vi "Control & Mapping.vi"() -> ()   [LabVIEW 2015]
uses:
  <vilib>/Instr/_visa.llb/VISA Configure Serial Port (Instr).vi
  <vilib>/Utility/inputDevices.llb/keyboardAcquire.vi
  <vilib>/Utility/inputDevices.llb/closeKeyboard.vi
panel:
  in  "path to PNG file":path
  out "Metres Travelled":dbl
  out "From Xbee":string
  out "Metal Sensors":string
  out "yplot2":dbl
  out "xplot2":dbl
  out "yplot1":dbl
  out "xplot1":dbl
  out "Right MS":bool
  out "Left MS":bool
  out "hi":dbl
  out "Y":dbl
  out "X":dbl
  in  "Direction in the Field":dbl
  out "TR":bool
  out "TL":bool
  out "MAP (19x19)":picture
  out "R":bool
  out "B":bool
  out "L":bool
  out "F":bool
  out "To Xbee":string
  in  "Required Speed":dbl=1.0 min=1.0 max=3.0 step=1.0
  # "Note:\n1 --> Low Speed\n2 --> Medium Speed\n3 --> High Speed"
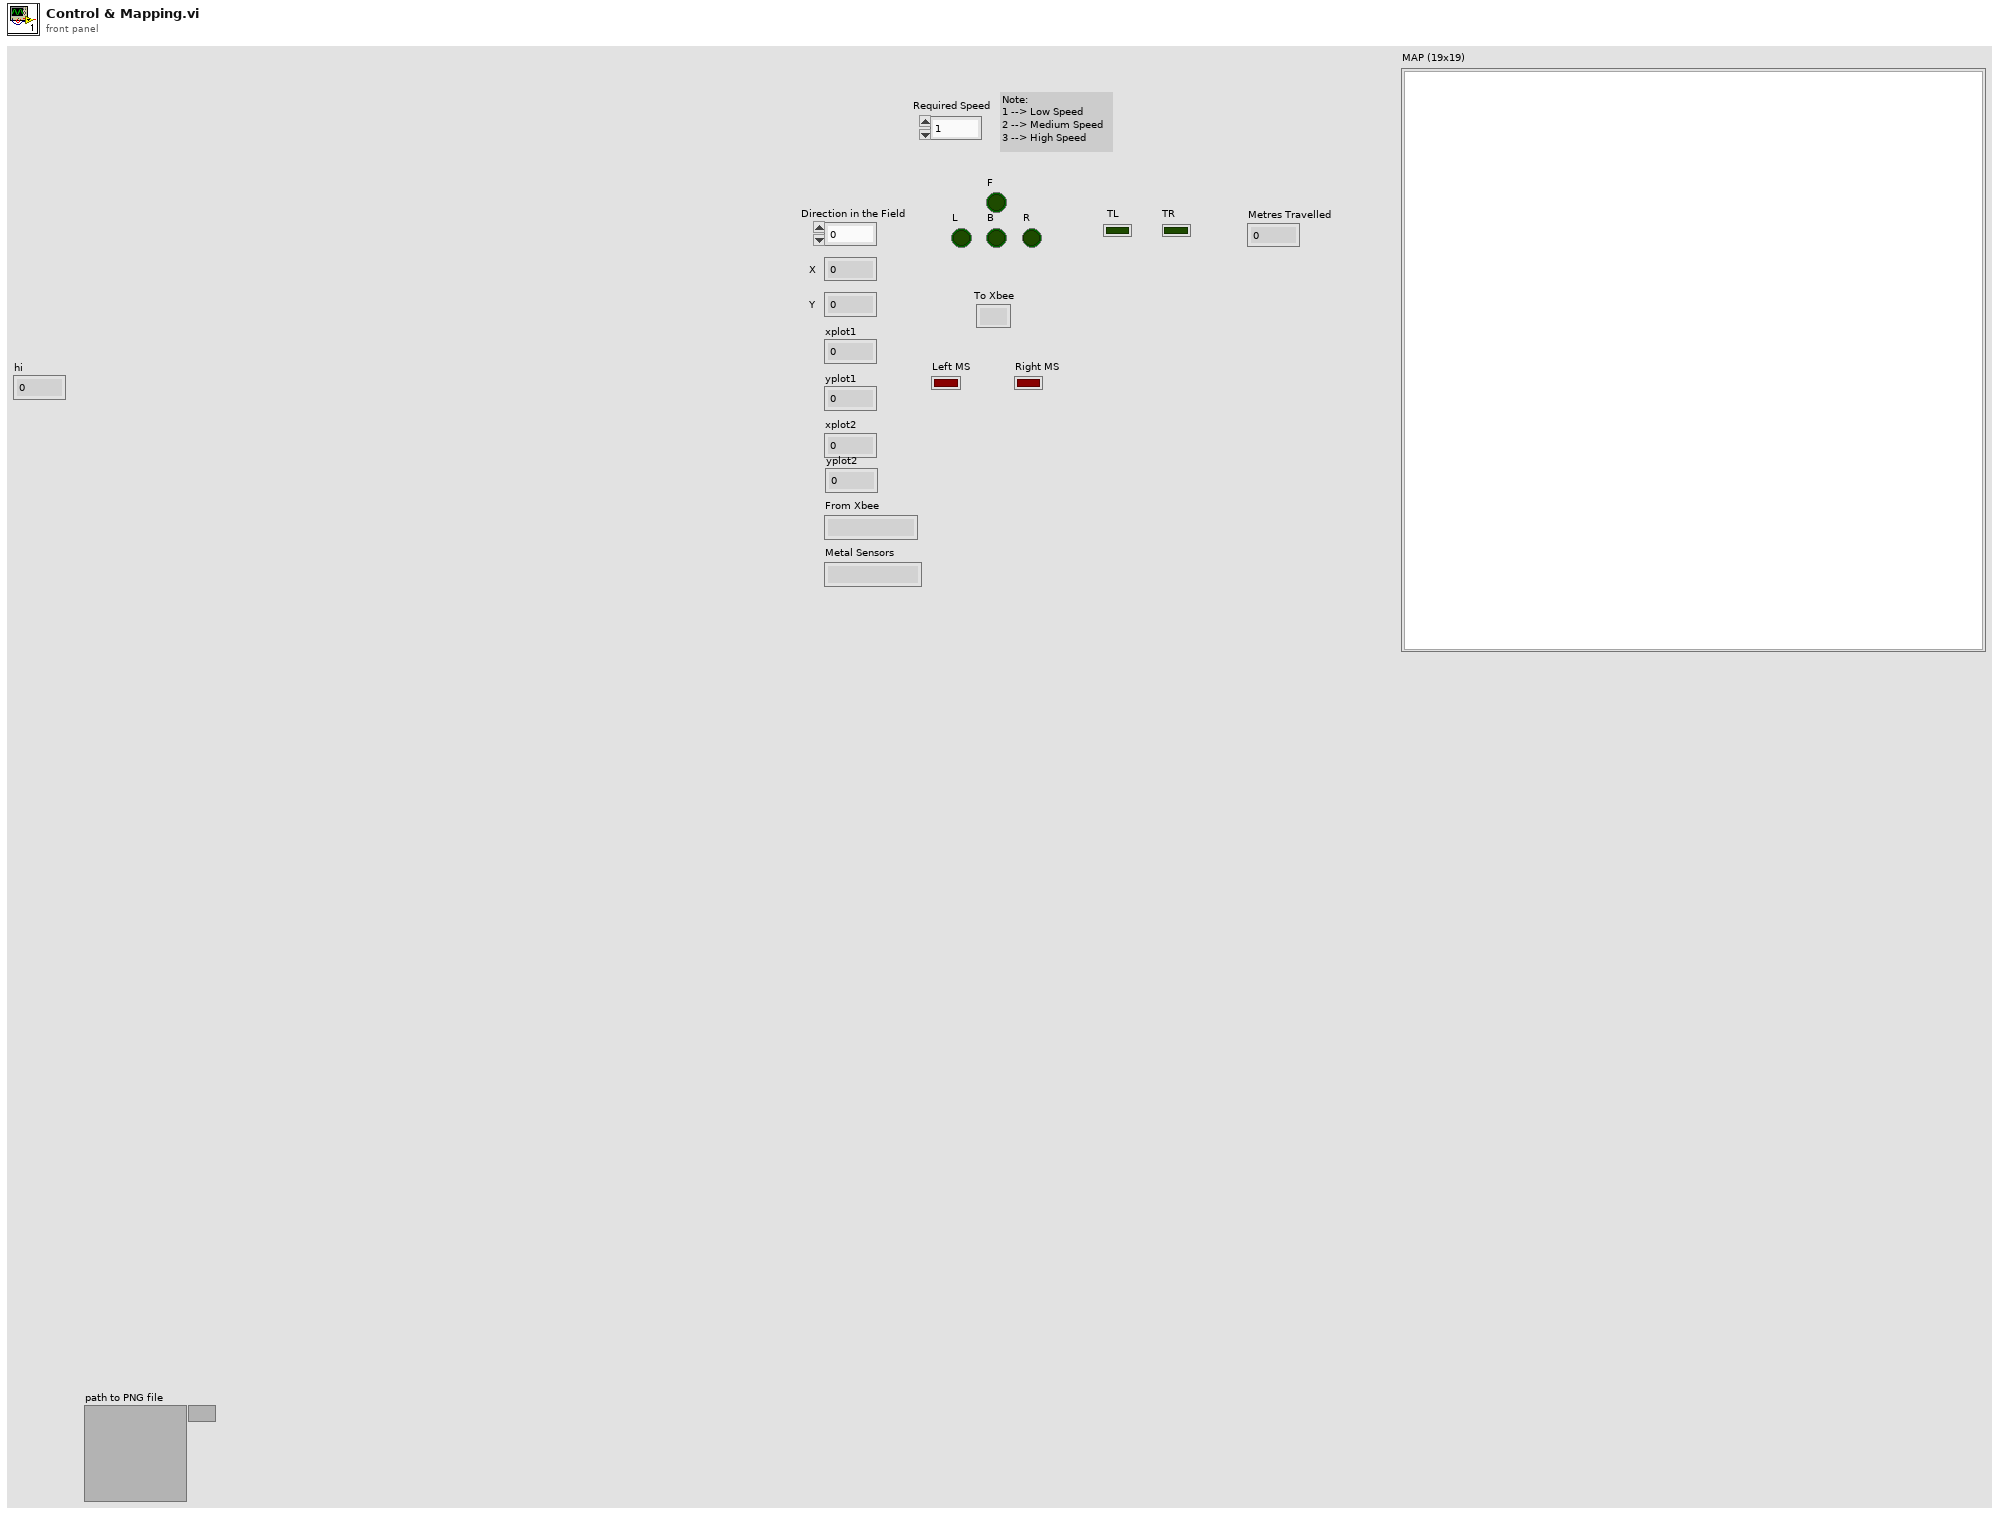
[diagram p1: front panel]
types:
  T1 = typedef "imagedata.ctl" = cluster{"image type":i32, "image depth":i32, "image":u8[], "mask":u8[], "colors":u32[], "Rectangle":cluster{"left":i16, "top":i16, "right":i16, "bottom":i16}}
  T2 = cluster{"Width":u16, "Style":enum32{"Solid", "Dash", "Dot", "DashDot", "DashDotDot"}}
  T3 = enum16{"0", "1", "2", "3", "4", "5", "6", "7", "8", "9", "A", "B", "C", "D", "E", "F", "G", "H", "I", "J", "K", "L", "M", "N", "O", "P", "Q", "R", "S", "T", "U", "V", "W", "X", "Y", "Z", "F1", "F2", "F3", "F4", "F5", "F6", "F7", "F8", "F9", "F10", "F11", "F12", "F13", "F14", "F15", "ADD", "BACK", "BACKSLASH", "CAPITAL", "COMMA", "DECIMAL", "DELETE", "DIVIDE", "DOWN", "END", "EQUALS", "ESCAPE", "GRAVE (`)", "HOME", "INSERT", "LBRACKET", "LCONTROL", "LEFT", "L ALT", "LSHIFT", "LWIN", "MINUS", "MULTIPLY", "NEXT", "NUMLOCK", "NUMPAD_0", "NUMPAD_1", "NUMPAD_2", "NUMPAD_3", "NUMPAD_4", "NUMPAD_5", "NUMPAD_6", "NUMPAD_7", "NUMPAD_8", "NUMPAD_9", "PAUSE", "PERIOD", "PRIOR (PG UP)", "RBRACKET", "RCONTROL", "RETURN", "RIGHT", "R ALT", "RSHIFT", "RWIN", "SCROLL", "SEMICOLON", "SLASH", "SPACE", "SUBTRACT", "TAB", "UP", "ENTER (num pad)", "' (quote)"}[]
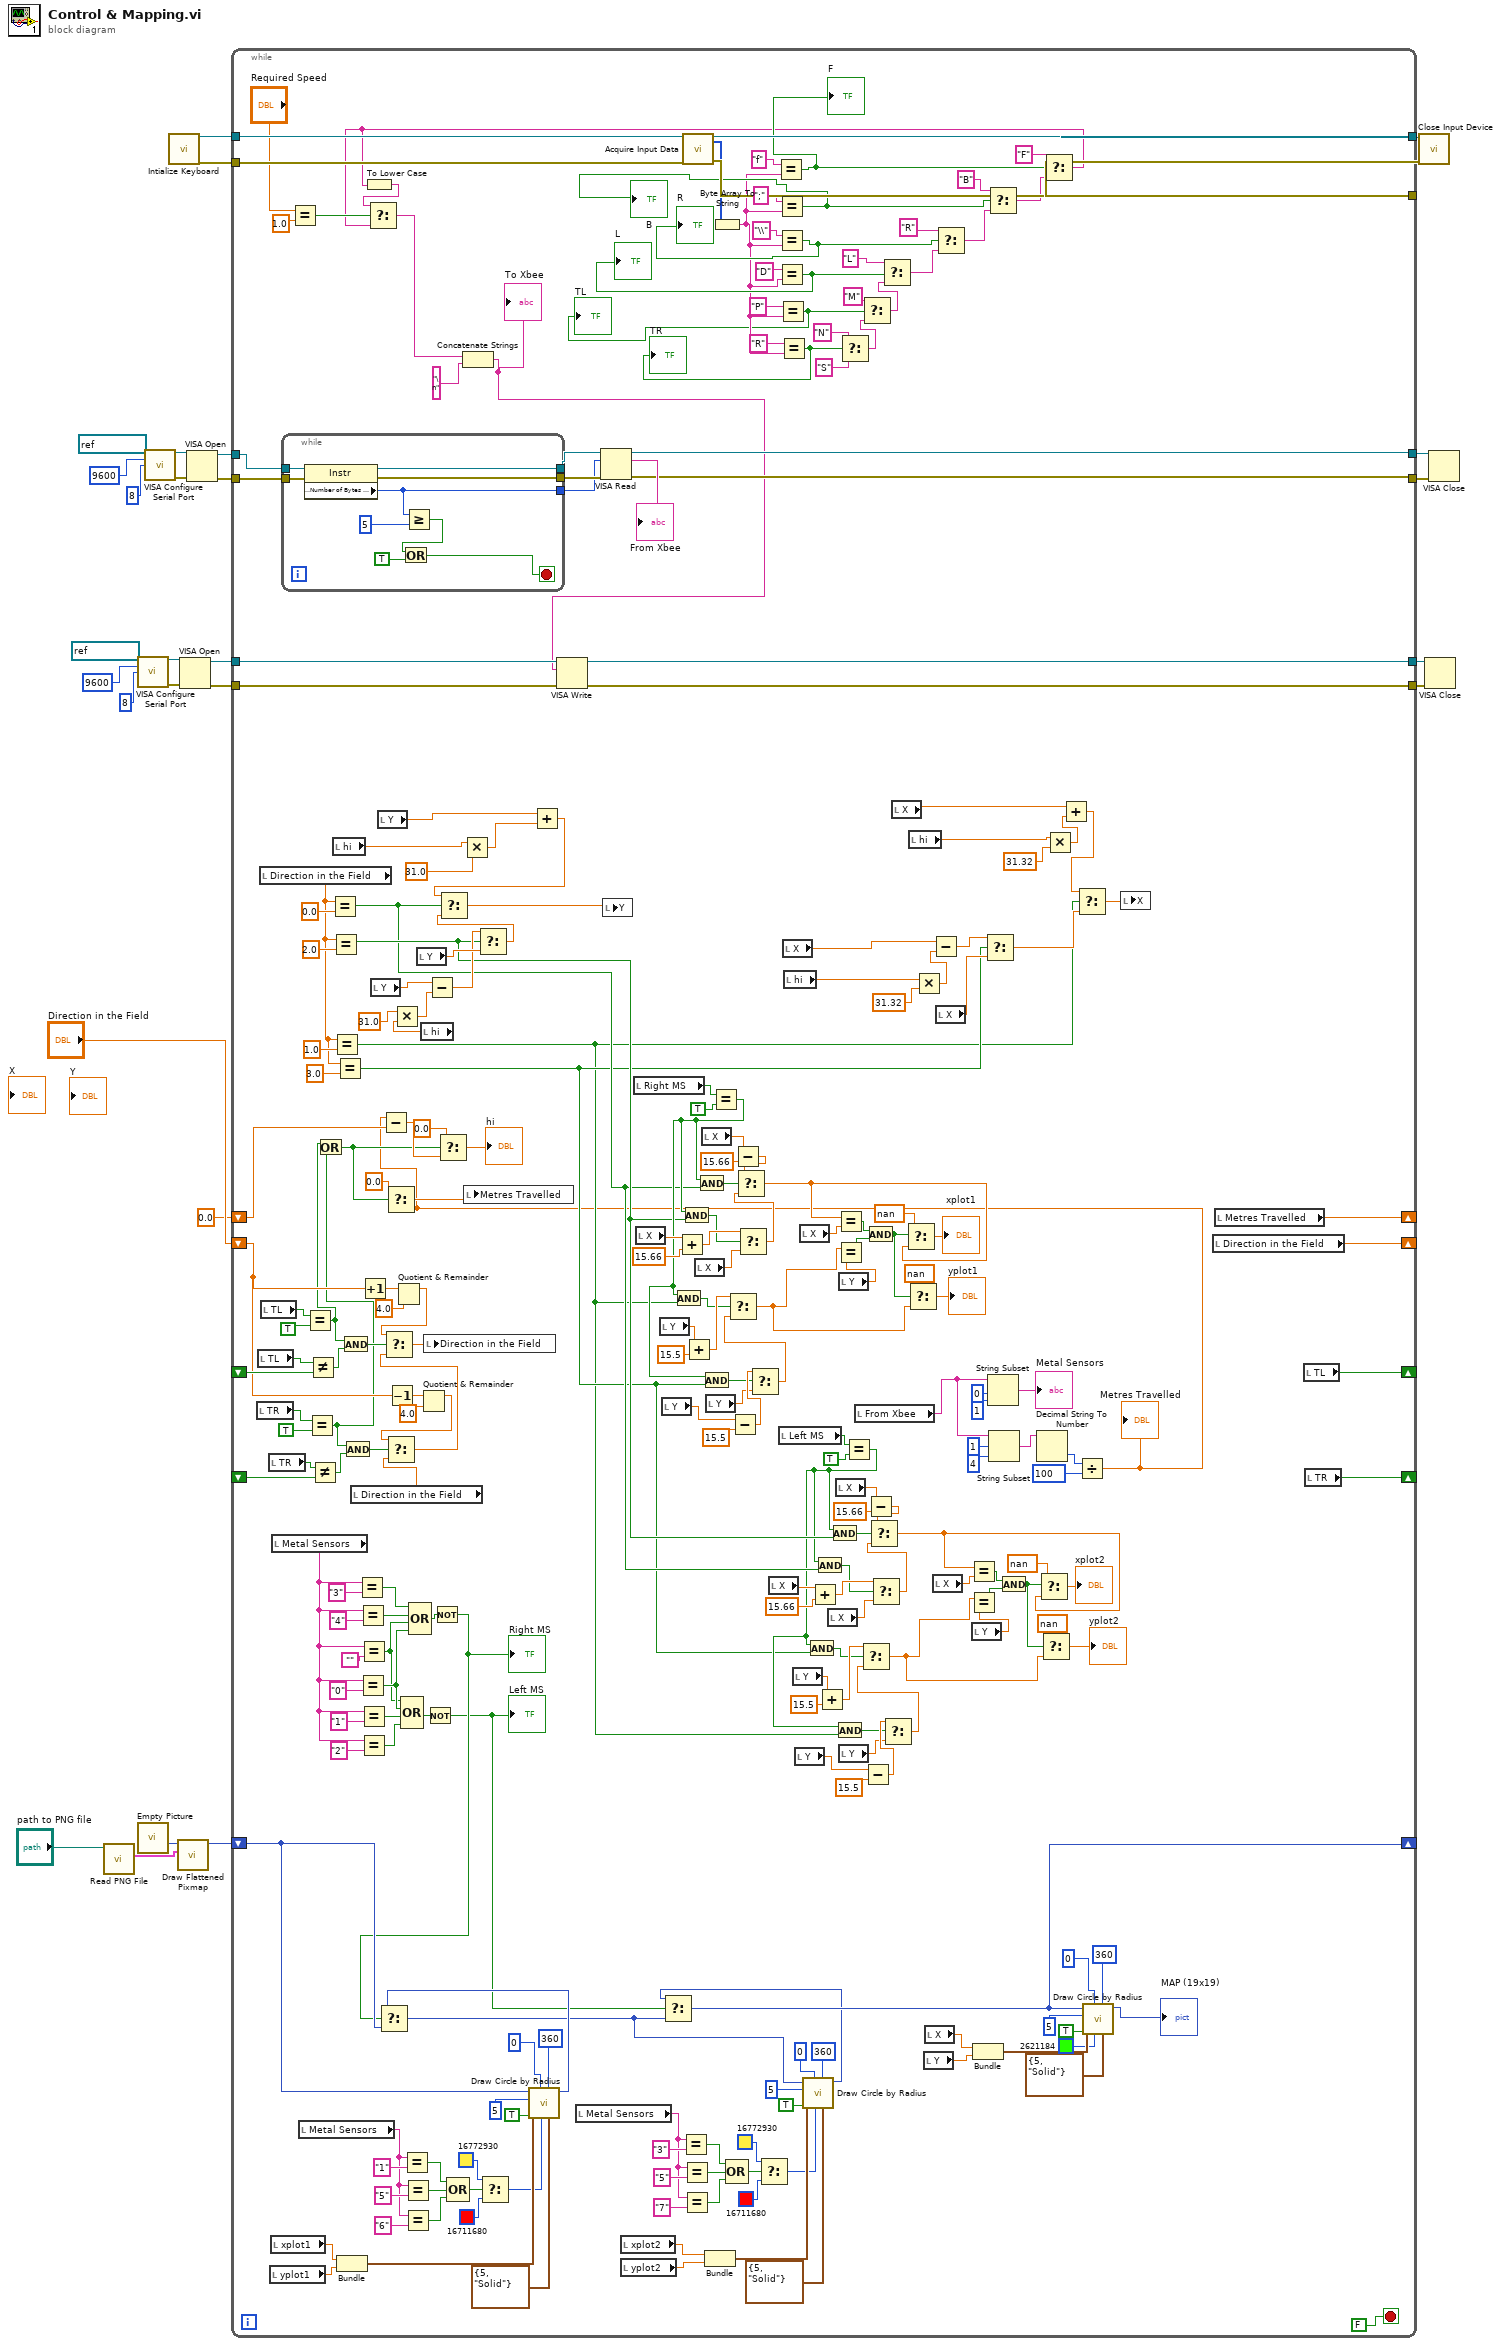
[diagram p0: block diagram]
diagram:
  n1 = call <vilib>:"Read PNG File.vi"("path to PNG file"="path to PNG file") -> ("image data"=w12:T1)  [unwired: 8 in, 2 out]
  n2 = call-poly "VISA Configure Serial Port"("VISA resource name"=refnum<visa-resource-name> "COM10", "baud rate (9600)"=u32 9600, "data bits (8)"=u16 8) -> ("VISA resource name out"=w9:refnum<visa-resource-name>, "error out"=w8:errorcluster)  [unwired: 11 in]
  n3 = call "Empty Picture"() -> ("empty picture"=w13:picture)
  n4 = call-poly "VISA Configure Serial Port"("VISA resource name"=refnum<visa-resource-name> "COM12", "baud rate (9600)"=u32 9600, "data bits (8)"=u16 8) -> ("VISA resource name out"=w20:refnum<visa-resource-name>, "error out"=w19:errorcluster)  [unwired: 11 in]
  n5 = call <vilib>:"Intialize Keyboard.vi"() -> ("error out"=w27:errorcluster, "device ID"=w28:refnum<k1>)  [unwired: 10 in]
  n6 = call <vilib>:"Draw Flattened Pixmap.vi"("image data"=w12, "picture"=w13) -> ("new picture"=w10:picture)  [unwired: 7 in]
  n7 = VISA Open(error in (no error)=w8, VISA resource name=w9) -> (VISA resource name=w4:refnum<visa-resource-name>, error out=w3:errorcluster)  [unwired: 3 in]
  n8 = VISA Open(error in (no error)=w19, VISA resource name=w20) -> (VISA resource name=w24:refnum<visa-resource-name>, error out=w21:errorcluster)  [unwired: 3 in]
  n9 = while {
    tunnel: w28 -> [w297]
    tunnel: w27 -> [w296]
    tunnel: [w295] -> w26
    tunnel: [w294] -> w25
    tunnel: w24 -> [w46]
    tunnel: [w35] -> w23
    tunnel: [w34] -> w22
    tunnel: w21 -> [w44]
    shift-right: [w226] -> _
    shift-left: 0.0 ("Metres Travelled (From Encoder)") -> [w197]
    shift-right: [w225] -> _
    shift-left: "Direction in the Field" -> [w202]
    shift-right: [w224] -> _
    shift-left: _ -> [w219]
    shift-right: [w223] -> _
    shift-left: _ -> [w211]
    shift-right: [w109] -> _
    shift-left: w10 -> [w165]
    tunnel: w4 -> [w33]
    tunnel: w3 -> [w32]
    tunnel: [w31] -> w2
    tunnel: [w30] -> w1
    stop <- FALSE stop-if-true
    n10 = local read "TR"() -> (w210:bool)
    n11 = local read "TL"() -> (w220:bool)
    n12 = local read "Direction in the Field"() -> (w231:dbl)
    n13 = local read "TL"() -> (w222:bool)
    n14 = local read "TR"() -> (w208:bool)
    n15 = local read "yplot1"() -> (w163:dbl)
    n16 = local read "xplot1"() -> (w162:dbl)
    n17 = local read "Metal Sensors"() -> (w40:string)
    n18 = while {
      tunnel: [w306] -> w43
      tunnel: w46 -> [w304]
      tunnel: [w303] -> w45
      tunnel: w44 -> [w302]
      tunnel: [w301] -> w42
      stop <- w298 stop-if-true
      n19 = property class="Instr"(reference=w304, error in=w302) -> (reference out=w303:refnum<visa-resource-name>, error out=w306:errorcluster, "Serial Settings:Number of Bytes at Serial Port"=w301:u32)
      n20 = Greater Or Equal?(x=w301, y=u32 5) -> (x >= y?=w300:bool)
      n21 = Or(x=w300, y=TRUE) -> (x .or. y?=w298:bool)
    }
    n22 = Equal?(x="Required Speed", y=1.0) -> (x = y?=w50:bool)
    n23 = local read "Metal Sensors"() -> (w81:string)
    n24 = Equal?(x=w222, y=TRUE) -> (x = y?=w36:bool)
    n25 = Equal?(x=w210, y=TRUE) -> (x = y?=w200:bool)
    n26 = Not Equal?(x=w220, y=w219) -> (x != y?=w218:bool)
    n27 = Not Equal?(x=w208, y=w211) -> (x != y?=w212:bool)
    n28 = Or(x=w36, y=w200) -> (x .or. y?=w195:bool)
    n29 = Equal?(x=w231, y=0.0) -> (x = y?=w113:bool)
    n30 = Equal?(x=w231, y=2.0) -> (x = y?=w114:bool)
    n31 = Equal?(x=w231, y=1.0) -> (x = y?=w110:bool)
    n32 = local read "hi"() -> (w253:dbl)
    n33 = Equal?(x=w231, y=3.0) -> (x = y?=w111:bool)
    n34 = Bundle("xplot1"=w162, "yplot1"=w163) -> (w171:cluster{"xplot1":dbl, "yplot1":dbl})  [unwired: 1 in]
    n35 = And(x=w36, y=w218) -> (x .and. y?=w217:bool)
    n36 = And(x=w200, y=w212) -> (x .and. y?=w207:bool)
    n37 = local read "Direction in the Field"() -> (w203:dbl)
    n38 = Equal?(x=w40, y="3") -> (x = y?=w95:bool)
    n39 = Equal?(x=w40, y="4") -> (x = y?=w94:bool)
    n40 = Equal?(x=w40, y="0") -> (x = y?=w41:bool)
    n41 = Equal?(x=w40, y="") -> (x = y?=w38:bool)
    n42 = Equal?(x=w40, y="1") -> (x = y?=w90:bool)
    n43 = Equal?(x=w40, y="2") -> (x = y?=w89:bool)
    n44 = Increment(x=w202) -> (x+1=w216:dbl)
    n45 = local read "Y"() -> (w236:dbl)
    n46 = local read "Y"() -> (w254:dbl)
    n47 = Decrement(x=w202) -> (x-1=w206:dbl)
    n48 = Quotient & Remainder(x=w216, y=4.0) -> (x-y*floor(x/y)=w214:dbl)  [unwired: 1 out]
    n49 = Compound Arithmetic op=OR(w38, w41, w90, w89) -> (w88:bool)
    n50 = Equal?(x=w81, y="1") -> (x = y?=w84:bool)
    n51 = Equal?(x=w81, y="5") -> (x = y?=w83:bool)
    n52 = Equal?(x=w81, y="6") -> (x = y?=w82:bool)
    n53 = Compound Arithmetic op=OR(w95, w94, w38, w41) -> (w93:bool)
    n54 = local read "Y"() -> (w235:dbl)
    n55 = Quotient & Remainder(x=w206, y=4.0) -> (x-y*floor(x/y)=w204:dbl)  [unwired: 1 out]
    n56 = Select(t=w204, s=w207, f=w203) -> (s? t:f=w201:dbl)
    n57 = Select(t=w214, s=w217, f=w201) -> (s? t:f=w213:dbl)
    n58 = local read "hi"() -> (w251:dbl)
    n59 = Multiply(x=31.0 ("y"), y=w251) -> (x*y=w249:dbl)
    n60 = local write "Direction in the Field"(w213) -> ()
    n61 = Not(x=w88) -> (.not. x?=w64:bool)
    "Left MS" <- w64
    n62 = Subtract(x=w236, y=w249) -> (x-y=w234:dbl)
    n63 = Not(x=w93) -> (.not. x?=w65:bool)
    "Right MS" <- w65
    n64 = Compound Arithmetic op=OR(w84, w83, w82) -> (w80:bool)
    n65 = Multiply(x=w253, y=31.0) -> (x*y=w252:dbl)
    n66 = Select(t=w234, s=w114, f=w235) -> (s? t:f=w233:dbl)
    n67 = Select(t=u32 16772930 ("color(black)"), s=w80, f=u32 16711680 ("color(black)")) -> (s? t:f=w77:u32)
    n68 = call <vilib>:"Draw Circle by Radius.vi"("pen"=T2 {"Width"=5, "Style"=enum."Solid"}, "arc size(360)"=360, "color(black)"=w77, "start angle(0)"=0, "fill?(F)"=TRUE, "pixel center"=w171, "radius"=i16 5, "picture"=w165) -> ("new picture"=w164:picture)  [unwired: 3 in]
    n69 = Select(t=w164, s=w65, f=w165) -> (s? t:f=w100:picture)
    n70 = Add(x=w254, y=w252) -> (x+y=w255:dbl)
    n71 = Select(t=w255, s=w113, f=w233) -> (s? t:f=w248:dbl)
    n72 = local read "Metal Sensors"() -> (w67:string)
    n73 = VISA Read(VISA resource name=w45, byte count=w42, error in (no error)=w43) -> (VISA resource name out=w35:refnum<visa-resource-name>, read buffer=→"From Xbee":string, error out=w34:errorcluster)  [unwired: 1 out]
    n74 = local write "Y"(w248) -> ()
    n75 = local read "xplot2"() -> (w103:dbl)
    n76 = local read "yplot2"() -> (w102:dbl)
    n77 = local read "Right MS"() -> (w191:bool)
    n78 = local read "X"() -> (w187:dbl)
    n79 = local read "Y"() -> (w181:dbl)
    n80 = local read "Y"() -> (w176:dbl)
    n81 = Add(x=w187, y=15.66) -> (x+y=w185:dbl)
    n82 = Equal?(x=w67, y="3") -> (x = y?=w73:bool)
    n83 = Equal?(x=w67, y="5") -> (x = y?=w72:bool)
    n84 = Equal?(x=w67, y="7") -> (x = y?=w71:bool)
    n85 = call-poly <vilib>:"Acquire Input Data.vi"("device ID"=w297, "error in (no error)"=w296) -> ("device ID"=w295:refnum<k1>, "keys pressed"=w292:T3, "error out"=w294:errorcluster)  [unwired: 15 in]
    n86 = Add(x=w181, y=15.5) -> (x+y=w179:dbl)
    n87 = local read "X"() -> (w161:dbl)
    n88 = local read "X"() -> (w189:dbl)
    n89 = Bundle("xplot2"=w103, "yplot2"=w102) -> (w108:cluster{"xplot2":dbl, "yplot2":dbl})  [unwired: 1 in]
    n90 = local read "Y"() -> (w159:dbl)
    n91 = Equal?(x=w191, y=TRUE) -> (x = y?=w178:bool)
    n92 = And(x=w178, y=w110) -> (x .and. y?=w174:bool)
    n93 = And(x=w178, y=w114) -> (x .and. y?=w182:bool)
    n94 = And(x=w178, y=w113) -> (x .and. y?=w183:bool)
    n95 = And(x=w178, y=w111) -> (x .and. y?=w173:bool)
    n96 = Byte Array To String(unsigned byte array=w292) -> (string=w275:string)
    n97 = Compound Arithmetic op=OR(w73, w72, w71) -> (w70:bool)
    n98 = Subtract(x=w176, y=15.5) -> (x-y=w175:dbl)
    n99 = Subtract(x=w189, y=15.66) -> (x-y=w188:dbl)
    n100 = Select(t=w185, s=w182, f=w161) -> (s? t:f=w184:dbl)
    n101 = Select(t=w188, s=w183, f=w184) -> (s? t:f=w152:dbl)
    n102 = Select(t=w175, s=w173, f=w159) -> (s? t:f=w177:dbl)
    n103 = Select(t=w179, s=w174, f=w177) -> (s? t:f=w149:dbl)
    n104 = Select(t=u32 16772930 ("color(black)"), s=w70, f=u32 16711680 ("color(black)")) -> (s? t:f=w66:u32)
    n105 = local read "X"() -> (w145:dbl)
    n106 = Equal?(x="f", y=w275) -> (x = y?=w279:bool)
    "F" <- w279
    n107 = Equal?(x=";", y=w275) -> (x = y?=w278:bool)
    "B" <- w278
    n108 = Equal?(x="\\", y=w275) -> (x = y?=w277:bool)
    "R" <- w277
    n109 = Equal?(x="D", y=w275) -> (x = y?=w276:bool)
    "L" <- w276
    n110 = Equal?(x="P", y=w275) -> (x = y?=w267:bool)
    "TL" <- w267
    n111 = Equal?(x="R", y=w275) -> (x = y?=w266:bool)
    "TR" <- w266
    n112 = local read "Left MS"() -> (w118:bool)
    n113 = local read "X"() -> (w240:dbl)
    n114 = local read "hi"() -> (w241:dbl)
    n115 = local read "Y"() -> (w139:dbl)
    n116 = local read "Y"() -> (w135:dbl)
    n117 = local read "X"() -> (w156:dbl)
    n118 = call <vilib>:"Draw Circle by Radius.vi"("pen"=T2 {"Width"=5, "Style"=enum."Solid"}, "arc size(360)"=360, "color(black)"=w66, "start angle(0)"=0, "fill?(F)"=TRUE, "pixel center"=w108, "radius"=i16 5, "picture"=w100) -> ("new picture"=w99:picture)  [unwired: 3 in]
    n119 = Select(t=w99, s=w64, f=w100) -> (s? t:f=w109:picture)
    n120 = Add(x=w145, y=15.66) -> (x+y=w143:dbl)
    n121 = Add(x=w139, y=15.5) -> (x+y=w137:dbl)
    n122 = local read "X"() -> (w131:dbl)
    n123 = Equal?(x=w152, y=w156) -> (x = y?=w158:bool)
    n124 = local read "X"() -> (w117:dbl)
    n125 = local read "Y"() -> (w155:dbl)
    n126 = Equal?(x=w149, y=w155) -> (x = y?=w157:bool)
    n127 = local read "Y"() -> (w129:dbl)
    n128 = Select(t="N", s=w266, f="S") -> (s? t:f=w269:string)
    n129 = Equal?(x=w118, y=TRUE) -> (x = y?=w112:bool)
    n130 = And(x=w112, y=w111) -> (x .and. y?=w133:bool)
    n131 = And(x=w112, y=w113) -> (x .and. y?=w140:bool)
    n132 = And(x=w112, y=w114) -> (x .and. y?=w141:bool)
    n133 = And(x=w112, y=w110) -> (x .and. y?=w132:bool)
    n134 = local read "From Xbee"() -> (w55:string)
    n135 = Select(t="M", s=w267, f=w269) -> (s? t:f=w270:string)
    n136 = Subtract(x=w135, y=15.5) -> (x-y=w134:dbl)
    n137 = And(x=w158, y=w157) -> (x .and. y?=w151:bool)
    n138 = Subtract(x=w117, y=15.66) -> (x-y=w146:dbl)
    n139 = Select(t=w143, s=w140, f=w131) -> (s? t:f=w142:dbl)
    n140 = Select(t=w146, s=w141, f=w142) -> (s? t:f=w123:dbl)
    n141 = Select(t="L", s=w276, f=w270) -> (s? t:f=w285:string)
    n142 = Select(t=w134, s=w132, f=w129) -> (s? t:f=w136:dbl)
    n143 = Select(t=w137, s=w133, f=w136) -> (s? t:f=w120:dbl)
    n144 = local read "X"() -> (w244:dbl)
    n145 = Select(t=nan, s=w151, f=w152) -> (s? t:f=→"xplot1":dbl)
    n146 = Select(t=nan, s=w151, f=w149) -> (s? t:f=→"yplot1":dbl)
    n147 = local read "hi"() -> (w247:dbl)
    n148 = Multiply(x=w241, y=31.32) -> (x*y=w229:dbl)
    n149 = local read "Y"() -> (w237:dbl)
    n150 = local read "X"() -> (w238:dbl)
    n151 = Subtract(x=w240, y=w229) -> (x-y=w230:dbl)
    n152 = local read "X"() -> (w126:dbl)
    n153 = Select(t="R", s=w277, f=w285) -> (s? t:f=w287:string)
    n154 = local read "X"() -> (w228:dbl)
    n155 = Equal?(x=w123, y=w126) -> (x = y?=w128:bool)
    n156 = local read "Y"() -> (w125:dbl)
    n157 = Equal?(x=w120, y=w125) -> (x = y?=w127:bool)
    n158 = Bundle("X"=w238, "Y"=w237) -> (w265:cluster{"X":dbl, "Y":dbl})  [unwired: 1 in]
    n159 = Select(t=w230, s=w111, f=w228) -> (s? t:f=w227:dbl)
    n160 = Select(t="B", s=w278, f=w287) -> (s? t:f=w286:string)
    n161 = String Subset(string=w55, offset (0)=0, length (rest)=1 ("length (rest)")) -> (substring=→"Metal Sensors":string)
    n162 = String Subset(string=w55, offset (0)=1, length (rest)=4 ("length (rest)")) -> (substring=w58:string)
    n163 = And(x=w128, y=w127) -> (x .and. y?=w122:bool)
    n164 = Decimal String To Number(string=w58) -> (number=w57:i32)  [unwired: 2 in, 1 out]
    n165 = Select(t=nan, s=w122, f=w123) -> (s? t:f=→"xplot2":dbl)
    n166 = Select(t=nan, s=w122, f=w120) -> (s? t:f=→"yplot2":dbl)
    n167 = Select(t="F", s=w279, f=w286) -> (s? t:f=w48:string)
    n168 = To Lower Case(string=w48) -> (all lower case string=w49:string)
    n169 = Select(t=w49, s=w50, f=w48) -> (s? t:f=w47:string)
    n170 = Concatenate Strings(w47, "\n" ("string")) -> (w29:string)
    "To Xbee" <- w29
    n171 = VISA Write(VISA resource name=w33, write buffer=w29, error in (no error)=w32) -> (VISA resource name out=w31:refnum<visa-resource-name>, error out=w30:errorcluster)  [unwired: 1 out]
    n172 = Multiply(x=w247, y=31.32) -> (x*y=w245:dbl)
    n173 = Add(x=w244, y=w245) -> (x+y=w243:dbl)
    n174 = Select(t=w243, s=w110, f=w227) -> (s? t:f=w239:dbl)
    n175 = Divide(x=w57, y=100) -> (x/y=w37:dbl)
    "Metres Travelled" <- w37
    n176 = Subtract(x=w37, y=w197) -> (x-y=w196:dbl)
    n177 = Select(t=0.0, s=w195, f=w37) -> (s? t:f=w193:dbl)
    n178 = Select(t=0.0, s=w195, f=w196) -> (s? t:f=→"hi":dbl)
    n179 = local write "Metres Travelled"(w193) -> ()
    n180 = call <vilib>:"Draw Circle by Radius.vi"("pen"=T2 {"Width"=5, "Style"=enum."Solid"}, "arc size(360)"=360, "color(black)"=u32 2621184, "start angle(0)"=0, "fill?(F)"=TRUE, "pixel center"=w265, "radius"=i16 5, "picture"=w109) -> ("new picture"=→"MAP (19x19)":picture)  [unwired: 3 in]
    n181 = local write "X"(w239) -> ()
    n182 = local read "Direction in the Field"() -> (w225:dbl)
    n183 = local read "Metres Travelled"() -> (w226:dbl)
    n184 = local read "TL"() -> (w224:bool)
    n185 = local read "TR"() -> (w223:bool)
  }
  n186 = call-poly <vilib>:"Close Input Device.vi"("error in (no error)"=w25, "device ID"=w26) -> ()  [unwired: 8 in, 1 out]
  n187 = VISA Close(VISA resource name=w2, error in (no error)=w1) -> ()  [unwired: 1 out]
  n188 = VISA Close(VISA resource name=w23, error in (no error)=w22) -> ()  [unwired: 1 out]
